vi "Dialog.vi"(8 "error in (no error)":errorcluster, 11 "Limit":string) -> (0 "error out":errorcluster, 3 "true":bool)   [LabVIEW 2013]
panel:
  in  "OK Button":bool
  out "String":string
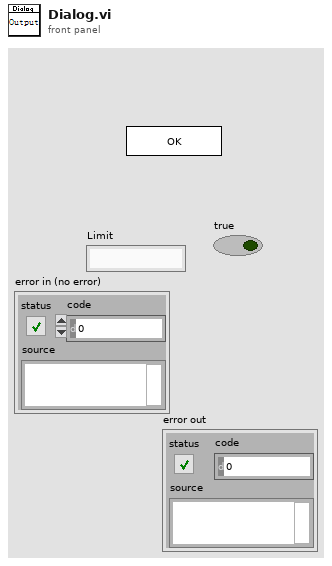
[diagram p1: front panel]
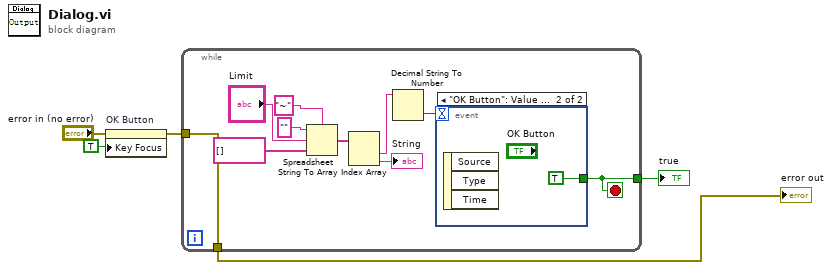
[diagram p0: block diagram]
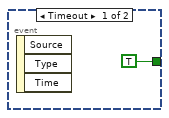
[diagram p2: hidden frame]
diagram:
  n1 = property on="OK Button" class="Bool"(error in="error in (no error)", "Key Focus"=TRUE) -> (error out=w3:errorcluster)  [unwired: 1 in, 1 out]
  n2 = while {
    tunnel: [w15] -> w5
    tunnel: w3 -> [w6]
    tunnel: [w6] -> w1
    stop <- w15 stop-if-true
    n3 = Spreadsheet String To Array(delimiter (Tab)="~", format string="", spreadsheet string="Limit", array type (2D Dbl)=string[] []) -> (array=w13:string[])
    n4 = Index Array(array=w13) -> (element #1=w14:string, element #2=→"String":string)  [unwired: 2 in]
    n5 = Decimal String To Number(string=w14) -> (number=w7:i32)  [unwired: 2 in, 1 out]
    n6 = event shown="[1] \"OK Button\": Value Change" {
      selector: _ -> [_ _]
      dyn-events: _ -> [_ _]
      timeout: w7 -> [_ _]
      tunnel: [TRUE TRUE] -> w15
      event Timeout {
        n7 = event-data() -> ()  [unwired: 1 in, 3 out]
      }
      event "OK Button": Value Change {
        n8 = event-data() -> ()  [unwired: 1 in, 3 out]
      }
    }
  }
  "true" <- w5
  "error out" <- w1
